vi "All Serializers.vi"() -> (3 "All serializers":refnum<class "BlueSerializer.lvclass">[](array[class]))   [LabVIEW 2019, in "Sports Unit Tests.lvclass"]
uses:
  Sports Unit Tests.lvclass
  <userlib>/Blue Origin/BlueSerialization/BlueSerializer/BlueSerializer.lvclass
  <userlib>/Blue Origin/BlueJSONTextSerializer/Classes/BlueJSONTextSerializer/BlueJSONTextSerializer.lvclass
  C:/Program Files (x86)/National Instruments/LabVIEW 2019/user.lib/Blue Origin/BlueSerialization/BlueSerializer/BlueSerializer.lvclass
  <userlib>/Blue Origin/BlueTOMLSerializer/Classes/BlueTOMLSerializer/BlueTOMLSerializer.lvclass
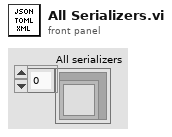
[diagram p1: front panel]
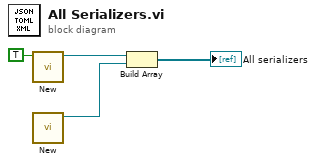
[diagram p0: block diagram]
diagram:
  n1 = call <userlib>:"New.vi"("PrettyPrint?"=TRUE) -> ("BlueJSONTextSerializer out"=w3:refnum<class "BlueJSONTextSerializer.lvclass">)  [unwired: 9 in, 1 out]
  n2 = call <userlib>:"New.vi"() -> ("BlueTOMLSerializer out"=w2:refnum<class "BlueTOMLSerializer.lvclass">)  [unwired: 10 in, 1 out]
  n3 = Build Array(w3, w2) -> (→"All serializers":refnum<class "BlueSerializer.lvclass">[])
